vi "SCMP - Write Eng Data v2.vi"(8 "error in":errorcluster, 9 "Temp Data":dbl[](array[numeric]), 10 "mesage":string) -> (0 "error out":errorcluster, 2 "Today's SCMP folder":path, 3 "first call":bool, 5 "Today's SCMP Engineering File":path)   [LabVIEW 2014]
doc: "This vi create or open file, which is save in format YYYYMMDD.txt. In this file are logs from CoMP-S Main program."
uses:
  Controls/Globals.vi
  Controls/Global demo.vi
panel:
  out "spreadsheet string":string
  out "Recent Log":string="\r"
  out "date/time string":string
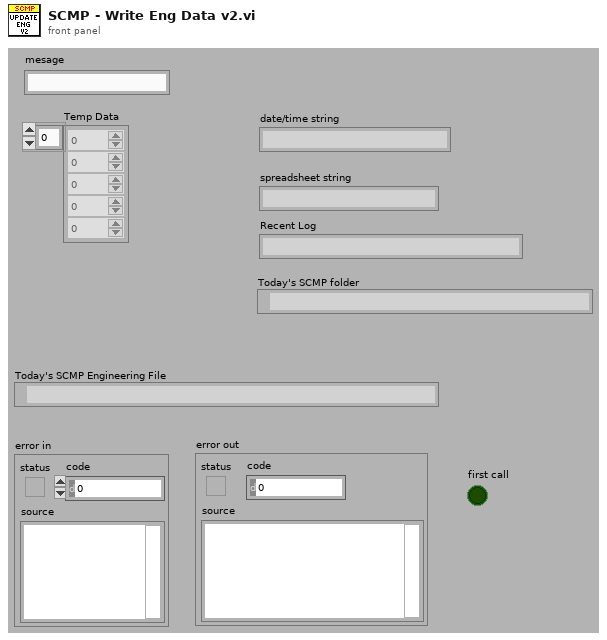
[diagram p1: front panel]
types:
  T1 = enum16{"open", "replace", "create", "open or create", "replace or create", "replace or create with confirmation"}
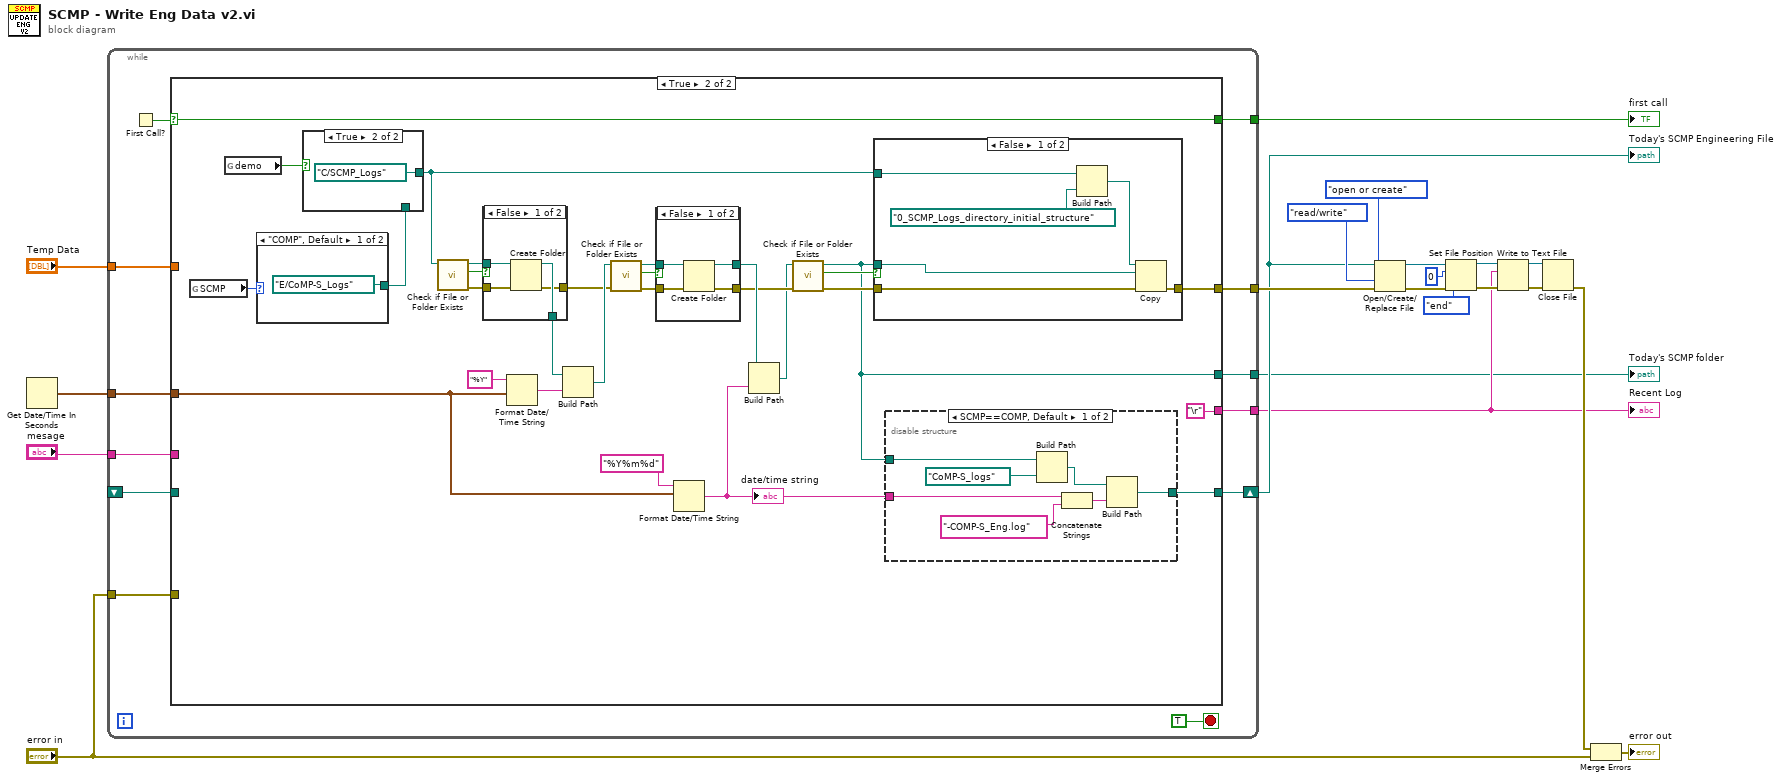
[diagram p0: block diagram]
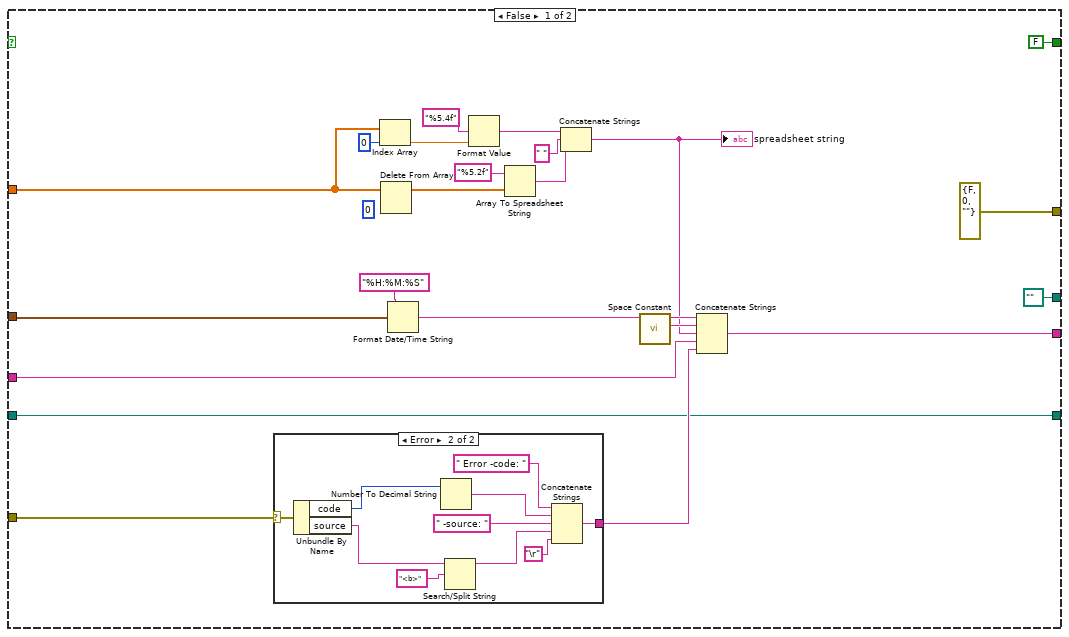
[diagram p2: hidden frame]
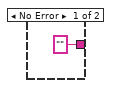
[diagram p3: hidden frame]
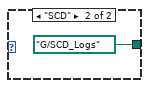
[diagram p4: hidden frame]
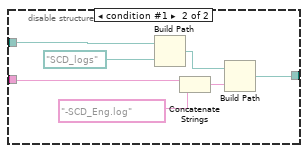
[diagram p6: hidden frame]
diagram:
  n1 = Get Date/Time In Seconds() -> (seconds since 1Jan1904=w17:timestamp)
  n2 = while {
    tunnel: w17 -> [w33]
    tunnel: "Temp Data" -> [w30]
    tunnel: "mesage" -> [w29]
    tunnel: "error in" -> [w28]
    tunnel: [w32] -> w16
    shift-right: [w26] -> w4
    shift-left: _ -> [w24]
    tunnel: [w25] -> w3
    tunnel: [w23] -> w2
    tunnel: [w22] -> w1
    stop <- TRUE stop-if-true
    n3 = First Call?() -> (First Call?: T/F=w31:bool)
    n4 = case shown="True" w31 {
      selector: w31 -> [_ w70]
      tunnel: w33 -> [w42 w77]
      tunnel: [errorcluster {"status"=FALSE, "code"=0, "source"=""} ("error out") w76] -> w32
      tunnel: w30 -> [w43 _]
      tunnel: w29 -> [w41 _]
      tunnel: w28 -> [w38 _]
      tunnel: [w36 w74] -> w26
      tunnel: [w37 "\r"] -> w25
      tunnel: w24 -> [w36 _]
      tunnel: [path "" ("dup path") w72] -> w23
      tunnel: [FALSE w70] -> w22
      frame False {
        (unwired) 0 ("index")
        n5 = case shown="Error" w38 {
          selector: w38 -> [_ w63]
          tunnel: ["" w61] -> w39
          frame No Error {
          }
          frame Error {
            n6 = Unbundle By Name(w63) -> ("code"=w62:i32, "source"=w58:string)
            n7 = Number To Decimal String(number=w62) -> (decimal integer string=w66:string)  [unwired: 1 in]
            n8 = Search/Split String(string=w58, search string/char (-)="<b>") -> (substring before match=w57:string)  [unwired: 1 in, 2 out]
            n9 = Concatenate Strings(" Error -code: ", w66, " -source: ", w57, "\r") -> (w61:string)
          }
        }
        n10 = Index Array(array=w43, index=0) -> (element=w47:dbl)
        n11 = Delete From Array(array=w43) -> (array with subset deleted=w45:dbl[])  [unwired: 2 in, 1 out]
        n12 = Format Date/Time String(time format string (%c)="%H:%M:%S", seconds (now)=w42) -> (date/time string=w52:string)  [unwired: 1 in]
        n13 = Format Value(format string="%5.4f", value (0)=w47) -> (output string=w49:string)  [unwired: 1 in]
        n14 = Array To Spreadsheet String(array=w45, 3:"%5.2f" ("format string")) -> (spreadsheet string=w50:string)  [unwired: 1 in]
        n15 = Concatenate Strings(w49, " " ("string"), w50) -> (w40:string)
        "spreadsheet string" <- w40
        n16 = call <vilib>:"Space Constant.vi"() -> ("String"=w53:string)
        n17 = Concatenate Strings(w52, w53, w40, w41, w39) -> (w37:string)
      }
      frame True {
        n18 = global read "Globals.vi" "SCMP"() -> (w68:enum16{"COMP", "SCD"})
        n19 = global read "Global demo.vi" "demo"() -> (w69:bool)
        n20 = case shown="\"COMP\", Default" w68 {
          tunnel: [path "E:/CoMP-S_Logs" ("Base SCMP Log File Folder") path "G:/SCD_Logs" ("Base SCMP Log File Folder")] -> w67
          frame "COMP", Default {
          }
          frame "SCD" {
          }
        }
        n21 = case shown="True" w69 {
          tunnel: [w97 path "C:/SCMP_Logs" ("Base SCMP Log File Folder")] -> w71
          tunnel: w67 -> [w97 _]
          frame False {
          }
          frame True {
          }
        }
        n22 = call <vilib>:"Check if File or Folder Exists.vi"("path"=w71) -> ("error out"=w83:errorcluster, "file or folder exists?"=w93:bool, "dup path"=w92:path)  [unwired: 8 in]
        n23 = case shown="False" w93 {
          tunnel: w92 -> [w129 w131]
          tunnel: [w128 w131] -> w89
          tunnel: [w127 w130] -> w85
          tunnel: w83 -> [w126 w130]
          frame False {
            n24 = Create Folder(path (use dialog)=w129, error in=w126) -> (created path=w128:path, error out=w127:errorcluster)  [unwired: 1 in, 1 out]
          }
          frame True {
          }
        }
        n25 = Format Date/Time String(time format string (%c)="%Y", seconds (now)=w77) -> (date/time string=w90:string)  [unwired: 1 in]
        n26 = Build Path(base path=w89, name or relative path=w90) -> (appended path=w86:path)
        n27 = call <vilib>:"Check if File or Folder Exists.vi"("error in (no error)"=w85, "path"=w86) -> ("error out"=w84:errorcluster, "file or folder exists?"=w88:bool, "dup path"=w87:path)  [unwired: 7 in]
        n28 = case shown="False" w88 {
          tunnel: w87 -> [w123 w124]
          tunnel: w84 -> [w122 w125]
          tunnel: [w121 w125] -> w79
          tunnel: [w120 w124] -> w80
          frame False {
            n29 = Create Folder(path (use dialog)=w123, error in=w122) -> (created path=w120:path, error out=w121:errorcluster)  [unwired: 1 in, 1 out]
          }
          frame True {
          }
        }
        n30 = Format Date/Time String(time format string (%c)="%Y%m%d", seconds (now)=w77) -> (date/time string=w75:string)  [unwired: 1 in]
        "date/time string" <- w75
        n31 = Build Path(base path=w80, name or relative path=w75) -> (appended path=w78:path)
        n32 = call <vilib>:"Check if File or Folder Exists.vi"("error in (no error)"=w79, "path"=w78) -> ("error out"=w82:errorcluster, "file or folder exists?"=w81:bool, "dup path"=w72:path)  [unwired: 7 in]
        n33 = case shown="False" w81 {
          tunnel: w72 -> [w113 _]
          tunnel: w82 -> [w115 w119]
          tunnel: w71 -> [w118 _]
          tunnel: [w114 w119] -> w76
          frame False {
            n34 = Build Path(base path=w118, name or relative path=path "0_SCMP_Logs_directory_initial_structure") -> (appended path=w116:path)
            n35 = Copy(8:w115, 10:w113, 11:w116) -> (0:w114:errorcluster)  [unwired: 2 in, 2 out]
          }
          frame True {
          }
        }
        n36 = disable-structure shown="SCMP==COMP, Default" {
          disable-tunnel: [w104 w108] -> w74
          disable-tunnel: w75 -> [w101 w107]
          disable-tunnel: w72 -> [w99 w106]
          frame condition #0 (active) {
            n37 = Build Path(base path=w99, name or relative path=path "CoMP-S_logs") -> (appended path=w102:path)
            n38 = Concatenate Strings(w101, "-COMP-S_Eng.log" ("string")) -> (w105:string)
            n39 = Build Path(base path=w102, name or relative path=w105) -> (appended path=w104:path)
          }
          frame condition #1 {
            n40 = Build Path(base path=w106, name or relative path=path "SCD_logs") -> (appended path=w110:path)
            n41 = Concatenate Strings(w107, "-SCD_Eng.log" ("string")) -> (w112:string)
            n42 = Build Path(base path=w110, name or relative path=w112) -> (appended path=w108:path)
          }
        }
      }
    }
  }
  "Today's SCMP Engineering File" <- w4
  "Recent Log" <- w3
  "Today's SCMP folder" <- w2
  "first call" <- w1
  n43 = Open/Create/Replace File(file path (use dialog)=w4, error in=w16, operation (0:open)=T1."open or create", access (0:read/write)=enum16{"read/write", "read-only", "write-only"}."read/write") -> (refnum out=w12:refnum<file>, error out=w13:errorcluster)  [unwired: 3 out]
  n44 = Set File Position(offset (in bytes) (0)=i64 0, refnum=w12, from (0:start)=enum16{"start", "end", "current"}."end", error in=w13) -> (refnum out=w21:refnum<file>, error out=w20:errorcluster)
  n45 = Write to Text File(file (use dialog)=w21, text=w3, error in=w20) -> (refnum out=w8:refnum<file>, error out=w9:errorcluster)  [unwired: 1 in, 1 out]
  n46 = Close File(refnum=w8, error in=w9) -> (error out=w18:errorcluster)  [unwired: 1 out]
  n47 = Merge Errors(w18, "error in") -> (→"error out":errorcluster)
